vi "StopData.vi"(8 "error in (no error)":errorcluster, 11 "RoomAlertIn":refnum<class "RoomAlert.lvclass">) -> (0 "error out":errorcluster, 3 "RoomAlertOut":refnum<class "RoomAlert.lvclass">)   [LabVIEW 2018, in "SensorPlugins.lvlib" / "RoomAlert.lvclass"]
uses:
  RoomAlert.lvclass
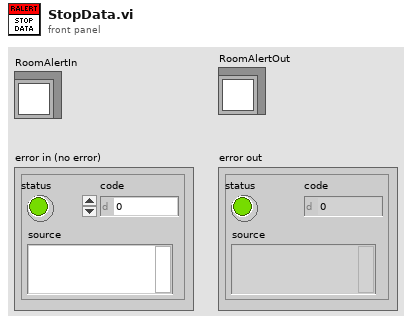
[diagram p1: front panel]
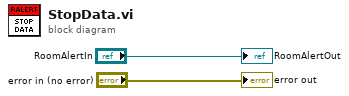
[diagram p0: block diagram]
diagram:
  "RoomAlertOut" <- "RoomAlertIn"
  "error out" <- "error in (no error)"
